vi "make_headers.vi"(8 "Error in":errorcluster, 9 "Accept":string, 10 "Content-Type":string, 11 "Device In":T1) -> (0 "Error Out":errorcluster, 3 "Device Out":T1)   [LabVIEW 2019]
uses:
  <userlib>/Onshape/_SubVI/Cluster.ctl
  <userlib>/Onshape/_SubVI/SHA256/SHA256.lvlib
  <vilib>/Utility/SMTP/NI_SMTPEmail.lvlib
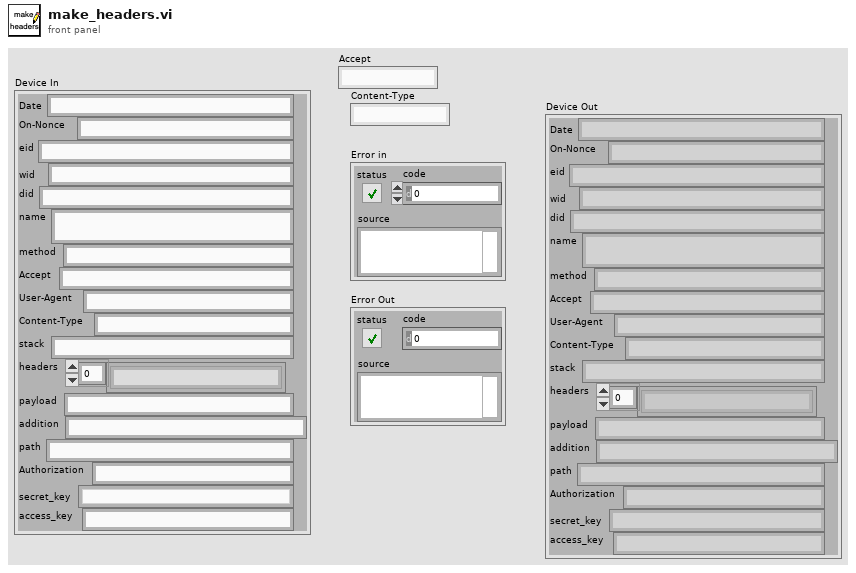
[diagram p1: front panel]
types:
  T1 = typedef "Cluster.ctl" = cluster{"Date":string, "On-Nonce":string, "eid":string, "wid":string, "did":string, "name":string, "method":string, "Accept":string, "User-Agent":string, "Content-Type":string, "stack":string, "headers":string[], "payload":string, "addition":string, "path":string, "Authorization":string, "secret_key":string, "access_key":string}
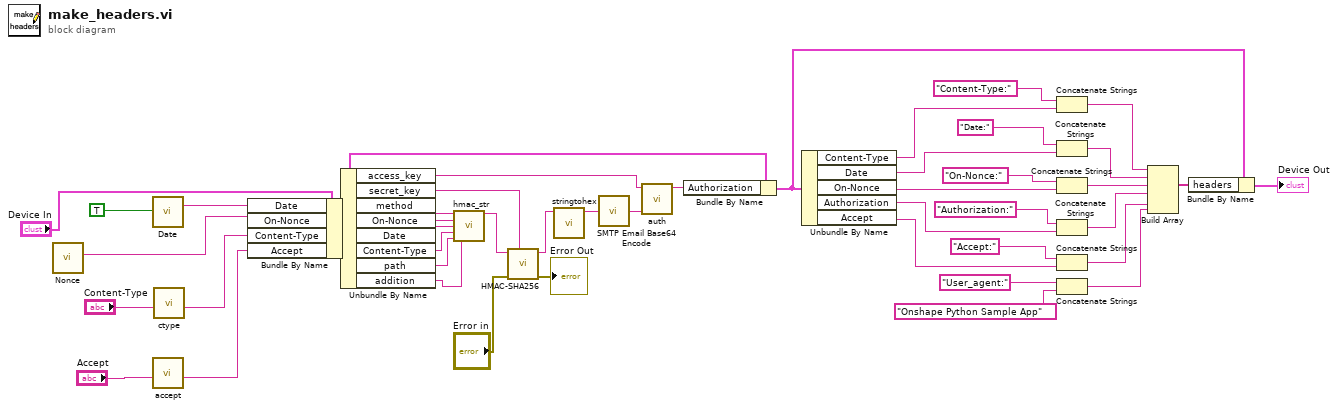
[diagram p0: block diagram]
diagram:
  n1 = call <userlib>:"Nonce.vi"() -> ("Nonce"=w1:string)  [unwired: 11 in]
  n2 = call <userlib>:"Date.vi"("UTC format"=TRUE) -> ("date/time string"=w33:string)  [unwired: 10 in]
  n3 = call <userlib>:"accept.vi"("Accept"="Accept") -> ("accept"=w11:string)  [unwired: 10 in]
  n4 = call <userlib>:"ctype.vi"("Content-Type"="Content-Type") -> ("ctype"=w44:string)  [unwired: 10 in]
  n5 = Bundle By Name(cluster="Device In", "Date"=w33, "On-Nonce"=w1, "Content-Type"=w44, "Accept"=w11) -> (w27:T1)
  n6 = Unbundle By Name(w27) -> ("access_key"=w34:string, "secret_key"=w35:string, "method"=w43:string, "On-Nonce"=w42:string, "Date"=w41:string, "Content-Type"=w39:string, "path"=w40:string, "addition"=w2:string)
  n7 = call <userlib>:"hmac_str.vi"("Method"=w43, "Nonce"=w42, "Date"=w41, "ctype"=w39, "path"=w40, "query"=w2) -> ("hmac_str"=w38:string)  [unwired: 9 in]
  n8 = call <userlib>:"HMAC-SHA256.vi"("Key"=w35, "error In"="Error in", "String to Encode"=w38) -> ("error Out"=→"Error Out":errorcluster, "Hash String"=w32:string)  [unwired: 7 in]
  n9 = call <userlib>:"stringtohex.vi"("Hash String"=w32) -> ("string"=w31:string)  [unwired: 10 in]
  n10 = call <userlib>:"SMTP Email Base64 Encode.vi"("Normal String"=w31) -> ("Base64 String"=w37:string)  [unwired: 1 in]
  n11 = call <userlib>:"auth.vi"("signature"=w37, "access_key"=w34) -> ("auth"=w36:string)  [unwired: 9 in]
  n12 = Bundle By Name(cluster=w27, "Authorization"=w36) -> (w26:T1)
  n13 = Unbundle By Name(w26) -> ("Content-Type"=w8:string, "Date"=w7:string, "On-Nonce"=w6:string, "Authorization"=w5:string, "Accept"=w4:string)
  n14 = Concatenate Strings("Content-Type:" ("string"), w8) -> (w20:string)
  n15 = Concatenate Strings("Date:" ("string"), w7) -> (w19:string)
  n16 = Concatenate Strings("On-Nonce:" ("string"), w6) -> (w18:string)
  n17 = Concatenate Strings("Authorization:" ("string"), w5) -> (w17:string)
  n18 = Concatenate Strings("Accept:" ("string"), w4) -> (w10:string)
  n19 = Concatenate Strings("User_agent:" ("string"), "Onshape Python Sample App" ("User-Agent")) -> (w9:string)
  n20 = Build Array(w20, w19, w18, w17, w10, w9) -> (w16:string[])
  n21 = Bundle By Name(cluster=w26, "headers"=w16) -> (→"Device Out":T1)
